vi "InitializeExpDepsFilesWithActualDeps.vi"() -> ()   [LabVIEW 2019, in "DepsWatch.lvlib"]
uses:
  <userlib>/_OpenG.lib/file/file.llb/File Exists - Scalar__ogtk.vi
  DepsWatch.lvlib
  <vilib>/Utility/config.llb/NI_LVConfig.lvlib
panel:
  out "ExpectedDeps Files Created":path[](array[path])
  out "error out":errorcluster
  in  "Build Specs Folder Path":path=path "C:/sw-deps-monitor/Source/BuildSpecs"
  in  "error in (no error)":errorcluster
  in  "Source Folder Path":path=path "C:/sw-deps-monitor/Source"
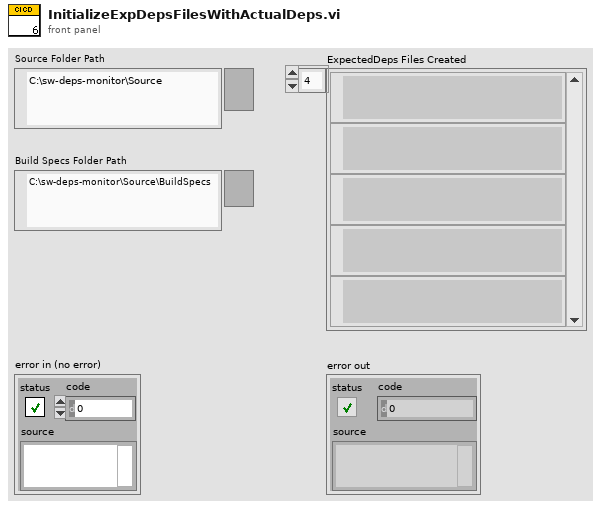
[diagram p1: front panel]
types:
  T1 = typedef "DepsWatch.lvlib/CICDPathConfigs.ctl" = cluster{"GlobalIncludePaths":path[], "GlobalExcludePaths":path[], "BuildSpecsIncludePaths":path[], "ActualDepsIncludePaths":path[], "WorkspacePath":path, "SourceFolderPaths":path[], "ChangedFilesLogpaths":map{string, path}}
  T2 = typedef "NI_LVConfig.lvlib/Config Data RefNum.ctl" = refnum<k1>
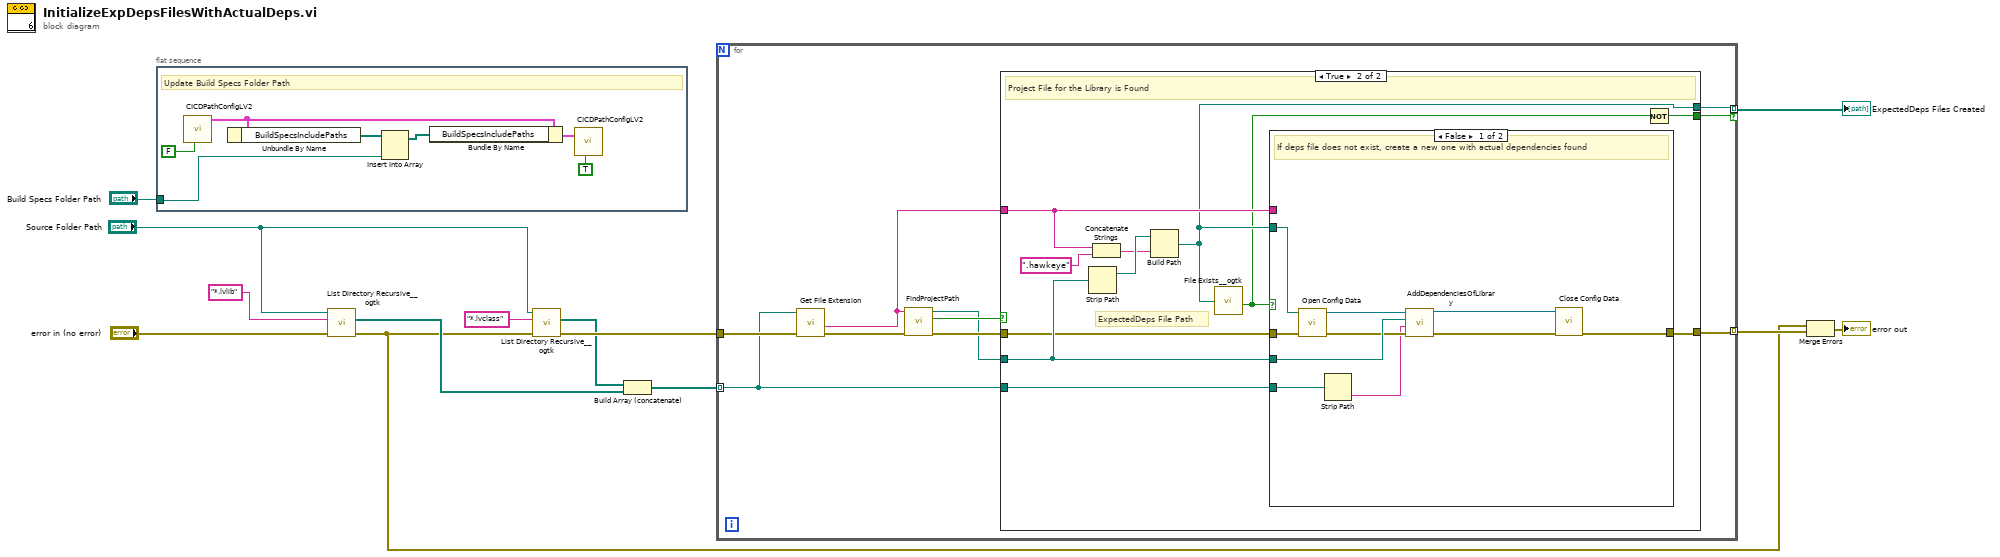
[diagram p0: block diagram]
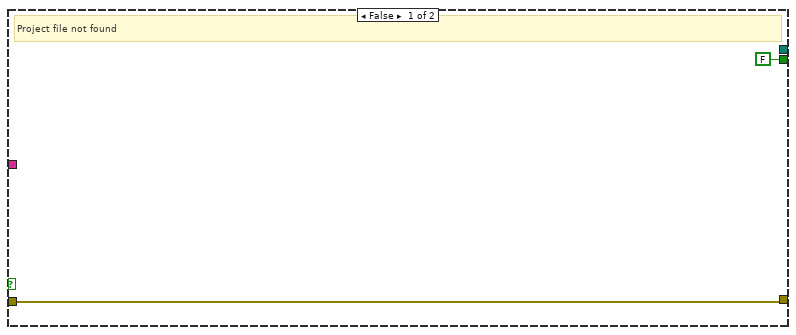
[diagram p2: hidden frame]
diagram:
  n1 = flat-sequence {
    tunnel: "Build Specs Folder Path" -> [w17]
    frame #0 {
      # "Update Build Specs Folder Path"
      n2 = call "CICDPathConfigLV2.vi"("Set? (F)"=FALSE) -> ("CICD Path Config Out"=w19:T1)  [unwired: 10 in]
      n3 = Unbundle By Name(w19) -> ("BuildSpecsIncludePaths"=w18:path[])
      n4 = Insert Into Array(array=w18, new element=w17) -> (w16:path[])  [unwired: 1 in]
      n5 = Bundle By Name(cluster=w19, "BuildSpecsIncludePaths"=w16) -> (w15:T1)
      n6 = call "CICDPathConfigLV2.vi"("Set? (F)"=TRUE, "CICD Path Config In"=w15) -> ()  [unwired: 9 in, 1 out]
    }
  }
  n7 = call <userlib>:"List Directory Recursive__ogtk.vi"("error in (no error)"="error in (no error)", "pattern"="*.lvlib", "Path"="Source Folder Path") -> ("error out"=w4:errorcluster, "file paths"=w11:path[])  [unwired: 5 in, 2 out]
  n8 = call <userlib>:"List Directory Recursive__ogtk.vi"("error in (no error)"=w4, "pattern"="*.lvclass", "Path"="Source Folder Path") -> ("error out"=w3:errorcluster, "file paths"=w1:path[])  [unwired: 5 in, 2 out]
  n9 = Build Array (concatenate)(w1, w11) -> (w2:path[])
  n10 = for {
    tunnel: w3 -> [w30]
    tunnel: w2 -> [w21] mode=indexing
    tunnel: [w29] -> w10 mode=indexing
    tunnel: [w24] -> w8 mode=indexing if=w23
    n11 = call <vilib>:"Get File Extension.vi"("error in (no error)"=w30, "file"=w21) -> ("error out"=w28:errorcluster, "filename without extension"=w22:string)  [unwired: 5 in, 3 out]
    n12 = call "FindProjectPath.vi"("error in (no error)"=w28, "Library/Class Name"=w22) -> ("error out"=w26:errorcluster, "Found?"=w27:bool, "Project Path"=w25:path)  [unwired: 7 in]
    n13 = case shown="True" w27 {
      tunnel: w26 -> [w32 w40]
      tunnel: w21 -> [_ w33]
      tunnel: [w32 w37] -> w29
      tunnel: w25 -> [_ w43]
      tunnel: w22 -> [_ w38]
      tunnel: [_ w36] -> w24
      tunnel: [FALSE w34] -> w23
      frame False {
        # "Project file not found"
      }
      frame True {
        # "ExpectedDeps File Path"
        # "Project File for the Library is Found"
        n14 = Strip Path(path=w43) -> (stripped path=w42:path)  [unwired: 1 out]
        n15 = Concatenate Strings(w38, ".hawkeye" ("string")) -> (w41:string)
        n16 = Build Path(base path=w42, name or relative path=w41) -> (appended path=w36:path)
        n17 = call-poly <userlib>:"File Exists__ogtk.vi"("file path"=w36) -> ("exists"=w35:bool)  [unwired: 6 in, 1 out]
        n18 = case shown="False" w35 {
          tunnel: w43 -> [w53 _]
          tunnel: w40 -> [w52 w54]
          tunnel: w36 -> [w51 _]
          tunnel: w38 -> [_ _]
          tunnel: [w46 w54] -> w37
          tunnel: w33 -> [w44 _]
          frame False {
            # "If deps file does not exist, create a new one with actual dependencies found"
            n19 = call <vilib>:"Open Config Data.vi"("error in (no error)"=w52, "configuration file path"=w51) -> ("error out"=w50:errorcluster, "refnum"=w49:T2)  [unwired: 7 in, 1 out]
            n20 = Strip Path(path=w44) -> (name=w45:string)  [unwired: 1 out]
            n21 = call "AddDependenciesOfLibrary.vi"("error in (no error)"=w50, "LibraryName"=w45, "Project Path"=w53, "Config Refnum in"=w49) -> ("error out"=w48:errorcluster, "Config Refnum out"=w47:T2)  [unwired: 4 in, 2 out]
            n22 = call <vilib>:"Close Config Data.vi"("error in (no error)"=w48, "refnum"=w47) -> ("error out"=w46:errorcluster)  [unwired: 8 in, 1 out]
          }
          frame True {
          }
        }
        n23 = Not(x=w35) -> (.not. x?=w34:bool)
      }
    }
  }
  "ExpectedDeps Files Created" <- w8
  n24 = Merge Errors(w4, w10) -> (→"error out":errorcluster)
